vi "Create LUT Key.vi"(9 "MD5":string, 10 "Caller VI Name":string) -> (2 "LUT Key":string)   [LabVIEW 2018, in "Assert API Components.lvlib" / "Process Monitor.lvlib"]
uses:
  Process Monitor.lvlib
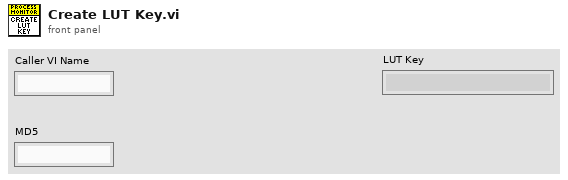
[diagram p1: front panel]
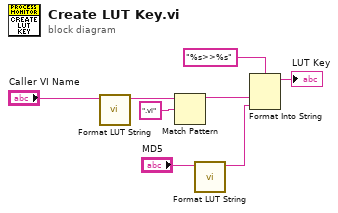
[diagram p0: block diagram]
diagram:
  n1 = call "Format LUT String.vi"("Input String"="Caller VI Name") -> ("Output String"=w3:string)  [unwired: 10 in]
  n2 = Match Pattern(string=w3, regular expression=".vi") -> (before substring=w1:string)  [unwired: 1 in, 3 out]
  n3 = call "Format LUT String.vi"("Input String"="MD5") -> ("Output String"=w6:string)  [unwired: 10 in]
  n4 = Format Into String(format string="%s>>%s", w1, w6) -> (resulting string=→"LUT Key":string)  [unwired: 2 in, 1 out]
